vi "Puff_Stats.vi"(6 "Puff release time (s)":dbl, 10 "Concentrations":dbl[](array[numeric]), 11 "Time (s)":dbl[](array[numeric])) -> (3 "Stats":dbl[](array[numeric]))   [LabVIEW 2012]
uses:
  <vilib>/Analysis/2dsp.llb/Integral Method.ctl
  <vilib>/Analysis/8numeric.llb/1D Numeric Integration.vi
  <vilib>/Analysis/NI_AALPro.lvlib
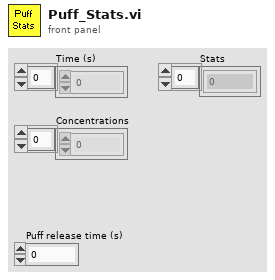
[diagram p1: front panel]
types:
  T1 = typedef "NI_AALPro.lvlib/Integral Method.ctl" = i32
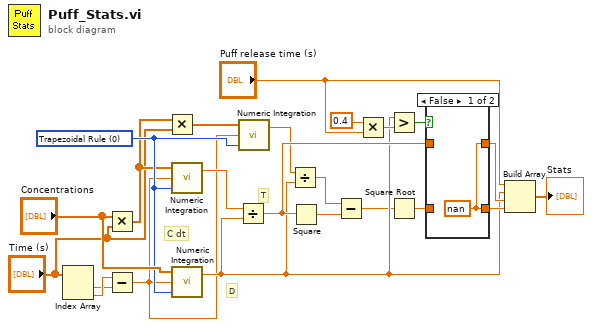
[diagram p0: block diagram]
diagram:
  w10 = T1 0 items=["Trapezoidal Rule", "Simpson's Rule", "Simpson's 3/8 Rule", "Bode Rule"] ("integration method")
  # "T"
  # "D"
  # "C dt"
  n1 = Index Array(array="Time (s)") -> (element #1=w2:dbl, element #2=w3:dbl)  [unwired: 2 in]
  n2 = Multiply(x="Concentrations", y="Time (s)") -> (x*y=w9:dbl[])
  n3 = Subtract(x=w3, y=w2) -> (x-y=w1:dbl)
  n4 = Multiply(x=w9, y="Time (s)") -> (x*y=w13:dbl[])
  n5 = call-poly <vilib>:"Numeric Integration.vi"("integration method"=w10, "dt"=w1, "Input Array"=w9) -> ("result"=w11:dbl)  [unwired: 1 out]
  n6 = call-poly <vilib>:"Numeric Integration.vi"("integration method"=w10, "dt"=w1, "Input Array"="Concentrations") -> ("result"=w14:dbl)  [unwired: 1 out]
  n7 = Divide(x=w11, y=w14) -> (x/y=w16:dbl)
  n8 = call-poly <vilib>:"Numeric Integration.vi"("integration method"=w10, "dt"=w1, "Input Array"=w13) -> ("result"=w12:dbl)  [unwired: 1 out]
  n9 = Divide(x=w12, y=w14) -> (x/y=w5:dbl)
  n10 = Square(x=w16) -> (x^2=w6:dbl)
  n11 = Subtract(x=w5, y=w6) -> (x-y=w7:dbl)
  n12 = Multiply(x=0.4 ("y"), y="Puff release time (s)") -> (x*y=w22:dbl)
  n13 = Greater?(x=w14, y=w22) -> (0:w15:bool)
  n14 = Square Root(x=w7) -> (sqrt(x)=w18:dbl)
  n15 = case shown="False" w15 {
    tunnel: [w24 w26] -> w17
    tunnel: w16 -> [_ w26]
    tunnel: [w24 w25] -> w19
    tunnel: w18 -> [_ w25]
    frame False {
      w24 = nan
    }
    frame True {
    }
  }
  n16 = Build Array("Puff release time (s)", w14, w17, w19) -> (→"Stats":dbl[])
